vi "Update RC Channel MAX MIN.vi"(8 "Error In":errorcluster, 11 "Aircraft ID":u8) -> (0 "error out":errorcluster)   [LabVIEW 2014]
uses:
  Aircraft Information/Controls/Aircraft RC Data.ctl
  Aircraft Information/Sub VI/Get Aircraft RC.vi
  Aircraft Information/Sub VI/Set Aircraft RC.vi
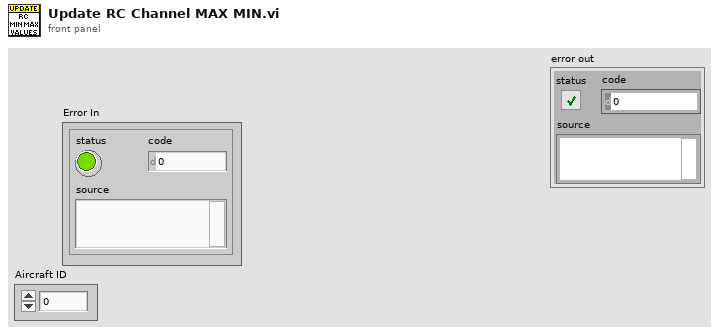
[diagram p1: front panel]
types:
  T1 = typedef "Aircraft RC Data.ctl" = cluster{"Channel 1 Min":i16, "Channel 1 Max":i16, "Channel 2 Min":i16, "Channel 2 Max":i16, "Channel 3 Min":i16, "Channel 3 Max":i16, "Channel 4 Min":i16, "Channel 4 Max":i16}
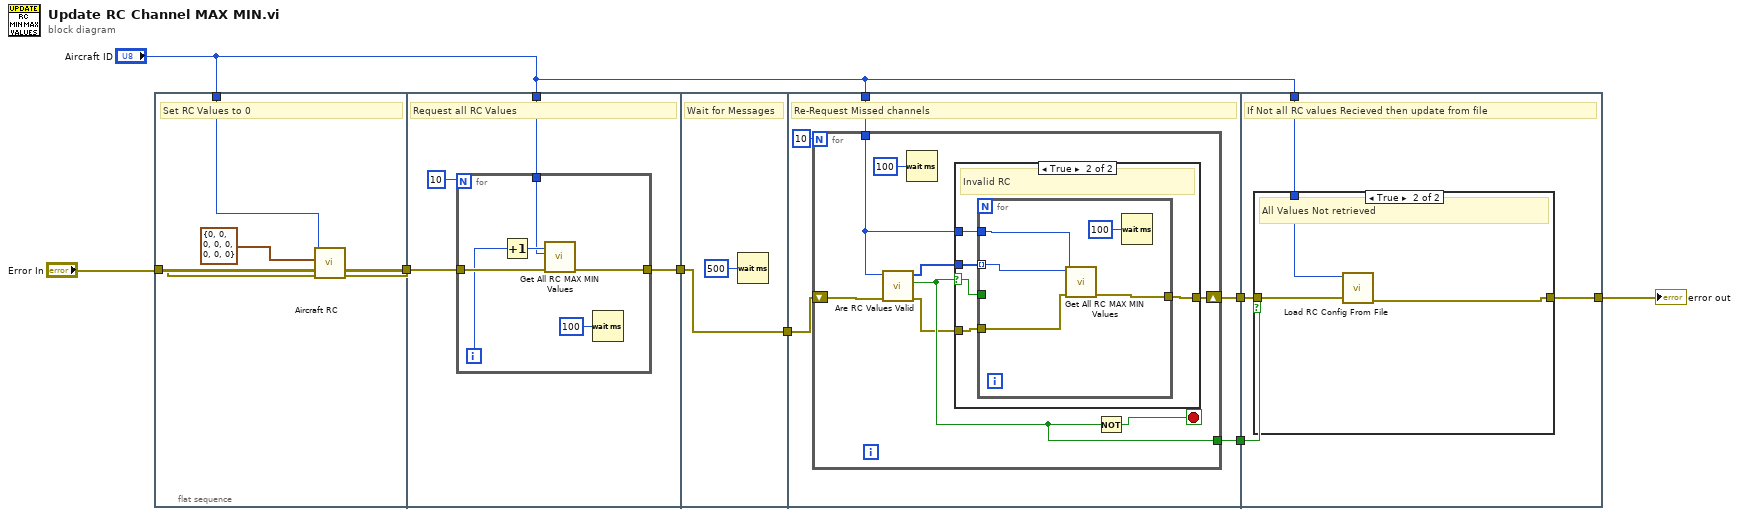
[diagram p0: block diagram]
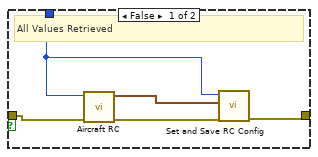
[diagram p3: hidden frame]
diagram:
  n1 = flat-sequence {
    tunnel: "Error In" -> [w11]
    tunnel: [w12] -> w2
    tunnel: "Aircraft ID" -> [w10]
    tunnel: [w14] -> w8
    tunnel: "Aircraft ID" -> [w13]
    tunnel: w2 -> [w15]
    tunnel: [w23] -> w7
    tunnel: w8 -> [w23]
    tunnel: w7 -> [w29]
    tunnel: [w28] -> w5
    tunnel: [w26] -> w4
    tunnel: "Aircraft ID" -> [w25]
    tunnel: w5 -> [w50]
    tunnel: w4 -> [w52]
    tunnel: [w51] -> w3
    tunnel: "Aircraft ID" -> [w49]
    frame #0 {
      # "Set RC Values to 0"
      n2 = call-poly "Aircraft RC.vi"("Error In"=w11, "Aircraft RC Data"=T1 {"Channel 1 Min"=0, "Channel 1 Max"=0, "Channel 2 Min"=0, "Channel 2 Max"=0, "Channel 3 Min"=0, "Channel 3 Max"=0, "Channel 4 Min"=0, "Channel 4 Max"=0}, "Aircraft ID"=w10) -> ("Error Out"=w12:errorcluster)  [unwired: 8 in]
    }
    frame #1 {
      # "Request all RC Values"
      n3 = for {
        N: 10 -> [_]
        tunnel: w15 -> [w22]
        tunnel: [w19] -> w14
        tunnel: w13 -> [w17]
        i -> [w20]
        n4 = Increment(x=w20) -> (x+1=w21:i32)
        n5 = call "Get All RC MAX MIN Values.vi"("error in (no error)"=w22, "Aircraft ID"=w17, "RC Channel"=w21) -> ("error out"=w19:errorcluster)  [unwired: 8 in]
        n6 = Wait (ms)(milliseconds to wait=u32 100) -> ()  [unwired: 1 out]
      }
    }
    frame #2 {
      # "Wait for Messages"
      n7 = Wait (ms)(milliseconds to wait=u32 500) -> ()  [unwired: 1 out]
    }
    frame #3 {
      # "Re-Request Missed channels"
      n8 = for {
        N: 10 -> [_]
        shift-right: [w36] -> w28
        shift-left: w29 -> [w32]
        tunnel: [w33] -> w26
        tunnel: w25 -> [w30]
        stop <- w34 stop-if-true
        n9 = call "Are RC Values Valid"("Error In"=w32, "Aircraft Index"=w30) -> ("Error Out"=w31:errorcluster, "RC Value Not Recieved"=w33:bool, "Unvalidated RC Channels"=w37:u16[])  [unwired: 7 in]
        n10 = Wait (ms)(milliseconds to wait=u32 100) -> ()  [unwired: 1 out]
        n11 = case shown="True" w33 {
          selector: w33 -> [_ w43]
          tunnel: w31 -> [w38 w42]
          tunnel: w37 -> [_ w41]
          tunnel: [w38 w40] -> w36
          tunnel: w30 -> [_ w39]
          frame False {
          }
          frame True {
            # "Invalid RC"
            n12 = for {
              tunnel: w43 -> [_]
              tunnel: w42 -> [w48]
              tunnel: w41 -> [w47] mode=indexing
              tunnel: [w46] -> w40
              tunnel: w39 -> [w45]
              n13 = call "Get All RC MAX MIN Values.vi"("error in (no error)"=w48, "Aircraft ID"=w45, "RC Channel"=w47) -> ("error out"=w46:errorcluster)  [unwired: 8 in]
              n14 = Wait (ms)(milliseconds to wait=u32 100) -> ()  [unwired: 1 out]
            }
          }
        }
        n15 = Not(x=w33) -> (.not. x?=w34:bool)
      }
    }
    frame #4 {
      # "If Not all RC values Recieved then update from file"
      n16 = case shown="True" w52 {
        tunnel: [w57 w58] -> w51
        tunnel: w50 -> [w55 w60]
        tunnel: w49 -> [w53 w59]
        frame False {
          # "All Values Retrieved"
          n17 = call-poly "Aircraft RC.vi"("Error In"=w55, "Aircraft ID"=w53) -> ("Error Out"=w56:errorcluster, "Aircraft RC Data"=w54:T1)  [unwired: 8 in]
          n18 = call "Set and Save RC Config.vi"("Error In"=w56, "Aircraft RC Data"=w54, "Aircraft Index"=w53) -> ("Error Out"=w57:errorcluster)  [unwired: 8 in]
        }
        frame True {
          # "All Values Not retrieved"
          n19 = call "Load RC Config From File.vi"("Error In"=w60, "Aircraft ID"=w59) -> ("Error Out"=w58:errorcluster)  [unwired: 9 in]
        }
      }
    }
  }
  "error out" <- w3
